vi "Get Key Names.vi"(7 "section":string, 8 "error in (no error)":errorcluster, 11 "refnum":T1) -> (0 "error out":errorcluster, 1 "key names":string[](array[string]), 2 "section exists?":bool, 3 "refnum out":T1)   [LabVIEW 2017, in "NI_LVConfig.lvlib"]
doc: "Gets the names of all keys in the specified section from the configuration data identified by <B>refnum</B>."
uses:
  <vilib>/Utility/config.llb/NI_LVConfig.lvlib
  <vilib>/Utility/config.llb/Config Data RefNum.ctl
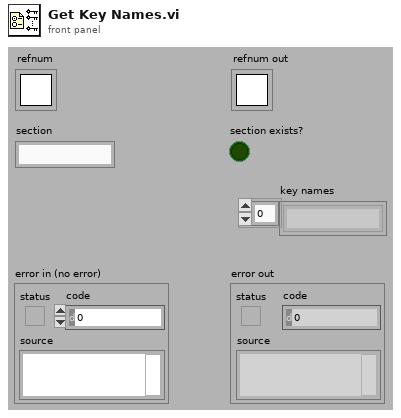
[diagram p1: front panel]
types:
  T1 = typedef "NI_LVConfig.lvlib/Config Data RefNum.ctl" = refnum<k1>
  T2 = typedef "NI_LVConfig.lvlib/Config Queue.ctl" = refnum<queue>
  T3 = typedef "NI_LVConfig.lvlib/Config Data.ctl" = cluster{"sections":T4[], "path":path, "dirty":bool}
  T4 = typedef "NI_LVConfig.lvlib/Section.ctl" = cluster{"name":string, "comment":string, "kvc":string[][]}
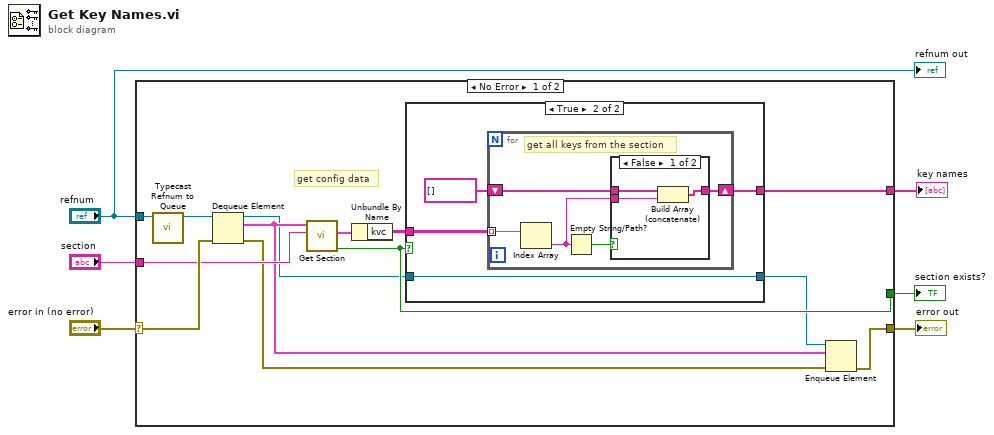
[diagram p0: block diagram]
diagram:
  n1 = case shown="No Error" "error in (no error)" {
    selector: "error in (no error)" -> [w16 w34]
    tunnel: [w13 _] -> w2
    tunnel: [w19 _] -> w1
    tunnel: [w10 w34] -> w4
    tunnel: "refnum" -> [w18 _]
    tunnel: "section" -> [w12 _]
    frame No Error {
      # "get config data"
      n2 = call <vilib>:"Typecast Refnum to Queue.vi"("refnum in"=w18) -> ("queue out"=w17:T2)  [unwired: 10 in]
      n3 = Dequeue Element(queue=w17, error in (no error)=w16) -> (queue out=w8:T2, element=w9:T3, error out=w11:errorcluster)  [unwired: 1 in, 1 out]
      n4 = call <vilib>:"Get Section.vi"("section"=w12, "element"=w9) -> ("section exists?"=w13:bool, "section data"=w15:T4)  [unwired: 6 in, 2 out]
      n5 = Unbundle By Name(w15) -> ("kvc"=w14:string[][])
      n6 = case shown="True" w13 {
        tunnel: [_ w23] -> w19
        tunnel: w14 -> [_ w24]
        tunnel: w8 -> [w20 w21]
        tunnel: [w20 w21] -> w7
        frame False {
        }
        frame True {
          n7 = for {
            tunnel: w24 -> [w29] mode=indexing
            shift-right: [w26] -> w23
            shift-left: string[] [] -> [w27]
            # "get all keys from the section"
            n8 = Index Array(array=w29) -> (element=w25:string)  [unwired: 1 in]
            n9 = Empty String/Path?(string/path=w25) -> (empty?=w28:bool)
            n10 = case shown="False" w28 {
              tunnel: w27 -> [w31 w33]
              tunnel: [w30 w33] -> w26
              tunnel: w25 -> [w32 _]
              frame False {
                n11 = Build Array (concatenate)(w31, w32) -> (w30:string[])
              }
              frame True {
              }
            }
          }
        }
      }
      n12 = Enqueue Element(queue=w7, element=w9, error in (no error)=w11) -> (error out=w10:errorcluster)  [unwired: 1 in, 2 out]
    }
    frame Error {
    }
  }
  "error out" <- w4
  "section exists?" <- w2
  "key names" <- w1
  "refnum out" <- "refnum"
